vi "Test Stamp Motion.vi"() -> ()   [LabVIEW 2011]
uses:
  Gantry Class/Gantry Class.lvclass
  GrabberTool Class.lvclass
panel:
  out "error out":errorcluster
  in  "Apply Stamp on Slot":i32
  in  "Apply Stamp on Chuck":i32
  in  "Stamp Slot":i32
  in  "Glue Reservoir Slot":i32
  in  "Config Folder":path=path "C:/Users/husker/Desktop/gantry/Config"
  in  "Virtual Mode":bool
  in  "Dip Stamp?":bool
  in  "Apply Stamp?":bool
  # "Defaults to Grab and Return Stamp\nCan also include Apply and Dip Stamp"
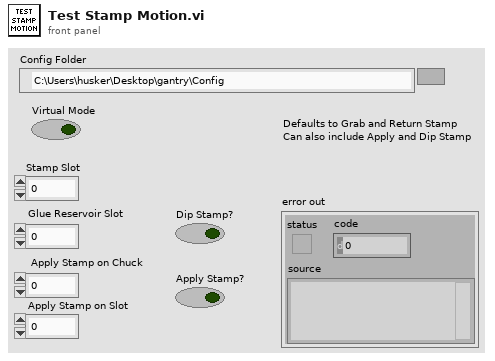
[diagram p1: front panel]
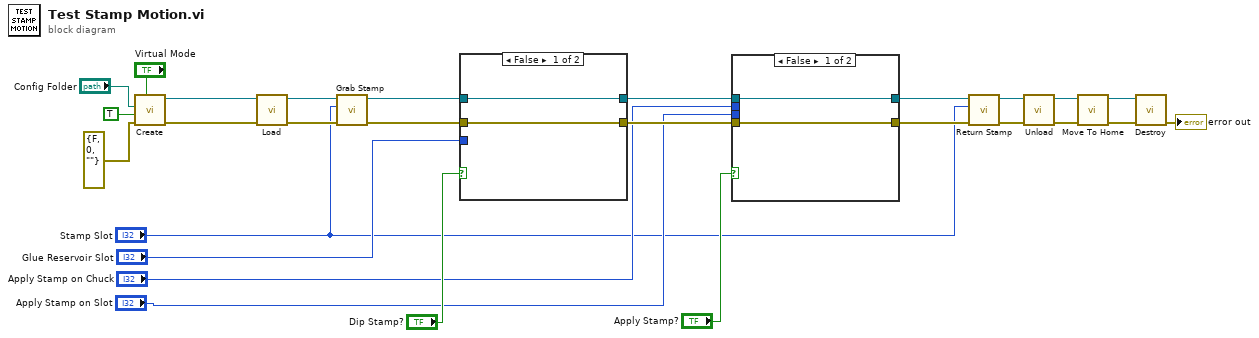
[diagram p0: block diagram]
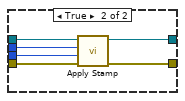
[diagram p2: hidden frame]
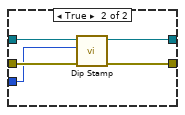
[diagram p3: hidden frame]
diagram:
  n1 = call "Create.vi"("Virtual Mode"="Virtual Mode", "error in"=errorcluster {"status"=FALSE, "code"=0, "source"=""}, "HOME?"=TRUE, "Config Folder"="Config Folder") -> ("error out"=w20:errorcluster, "Gantry out"=w21:refnum<class "Gantry Class.lvclass">)  [unwired: 6 in]
  n2 = call "Load.vi"("error in"=w20, "Gantry In"=w21) -> ("error out"=w18:errorcluster, "Grabber Tool out"=w19:refnum<class "GrabberTool Class.lvclass">)  [unwired: 8 in]
  n3 = call "Grab Stamp.vi"("error in"=w18, "Stamp Number"="Stamp Slot", "GrabberTool in"=w19) -> ("error out"=w16:errorcluster, "GrabberTool out"=w17:refnum<class "GrabberTool Class.lvclass">)  [unwired: 7 in]
  n4 = case shown="False" "Dip Stamp?" {
    tunnel: w17 -> [w29 w34]
    tunnel: w16 -> [w28 w33]
    tunnel: [w29 w32] -> w15
    tunnel: [w28 w31] -> w14
    tunnel: "Glue Reservoir Slot" -> [_ w30]
    frame False {
    }
    frame True {
      n5 = call "Dip Stamp.vi"("error in"=w33, "Reservoir Number"=w30, "GrabberTool in"=w34) -> ("error out"=w31:errorcluster, "GrabberTool out"=w32:refnum<class "GrabberTool Class.lvclass">)  [unwired: 7 in]
    }
  }
  n6 = case shown="False" "Apply Stamp?" {
    tunnel: w15 -> [w36 w42]
    tunnel: w14 -> [w35 w41]
    tunnel: [w36 w40] -> w13
    tunnel: [w35 w39] -> w12
    tunnel: "Apply Stamp on Chuck" -> [_ w38]
    tunnel: "Apply Stamp on Slot" -> [_ w37]
    frame False {
    }
    frame True {
      n7 = call "Apply Stamp.vi"("error in"=w41, "Slot Number"=w37, "Chuck Number"=w38, "GrabberTool in"=w42) -> ("error out"=w39:errorcluster, "GrabberTool out"=w40:refnum<class "GrabberTool Class.lvclass">)  [unwired: 6 in]
    }
  }
  n8 = call "Return Stamp.vi"("error in"=w12, "Slot Number"="Stamp Slot", "GrabberTool in"=w13) -> ("error out"=w10:errorcluster, "GrabberTool out"=w11:refnum<class "GrabberTool Class.lvclass">)  [unwired: 7 in]
  n9 = call "Unload.vi"("error in"=w10, "GrabberTool in"=w11) -> ("error out"=w8:errorcluster, "Gantry out"=w9:refnum<class "Gantry Class.lvclass">)  [unwired: 8 in]
  n10 = call-dynamic "Move To Home.vi"("error in"=w8, "Gantry in"=w9) -> ("error out"=w6:errorcluster, "Gantry out"=w7:refnum<class "Gantry Class.lvclass">)  [unwired: 8 in]
  n11 = call "Destroy.vi"("error in"=w6, "Gantry Class in"=w7) -> ("error out"=→"error out":errorcluster)  [unwired: 9 in]
